vi "PQerrorMessage.vi"(8 "error in (no error)":errorcluster, 11 "conn":u32) -> (0 "error out":errorcluster, 1 "PQerrorMessage":string, 3 "conn_out":u32)   [LabVIEW 2019, in "libpqlv.lvlib"]
doc: "Returns the error message most recently generated by an operation on the connection."
uses:
  libpqlv.lvlib
  libpq.dll
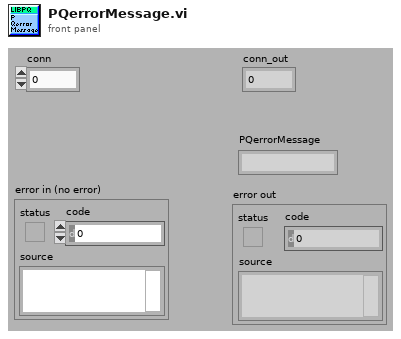
[diagram p1: front panel]
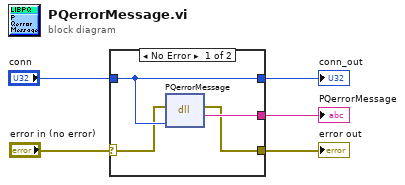
[diagram p0: block diagram]
diagram:
  n1 = case shown="No Error" "error in (no error)" {
    selector: "error in (no error)" -> [w7 w11]
    tunnel: [w6 w11] -> w4
    tunnel: [w9 _] -> w3
    tunnel: "conn" -> [w8 w10]
    tunnel: [w8 w10] -> w1
    frame No Error {
      n2 = dll-call lib="libpq.*" fn="PQerrorMessage"(error in=w7, "conn"=w8) -> (error out=w6:errorcluster, "PQerrorMessage"=w9:string)  [unwired: 3 in, 1 out]
    }
    frame Error {
    }
  }
  "PQerrorMessage" <- w3
  "error out" <- w4
  "conn_out" <- w1
